vi "List_Files.vi"(8 "error in (no error)":errorcluster, 11 "IB_Source_Container in":refnum<class "IB_Source_Container.lvclass">) -> (0 "error out":errorcluster, 3 "Files":T1[](array[typedef]))   [LabVIEW 2020, in "IB_Source_Container.lvclass"]
uses:
  <vilib>/AppBuilder/IB_Classes/Source/Container/IB_Source_Container.lvclass
  <vilib>/AppBuilder/IB_Classes/Source/Container/IB_Source_Container.lvclass/IB_Source_Container.ctl
  <vilib>/AppBuilder/IB_Classes/Source/IB_Source.lvclass
  <vilib>/AppBuilder/IB_Classes/Source/File/IB_Source_File.lvclass
  <resource>/Framework/Providers/Builds/Installer/CDK_sTypeDef_FileList.ctl
  e:/builds/penguin/labview/branches/2020/dev/dist/vi.lib/AppBuilder/IB_Classes/Source/IB_Source.lvclass
  e:/builds/penguin/labview/branches/2020/dev/dist/vi.lib/AppBuilder/IB_Classes/Source/Container/IB_Source_Container.lvclass
  <vilib>/AppBuilder/IB_Classes/Source/File/CtrFile/IB_CtrFile.lvclass
  e:/builds/penguin/labview/branches/2020/dev/dist/vi.lib/AppBuilder/IB_Classes/Source/File/IB_Source_File.lvclass
  e:/builds/penguin/labview/branches/2020/dev/dist/vi.lib/AppBuilder/IB_Classes/Source/File/CtrFile/IB_CtrFile.lvclass
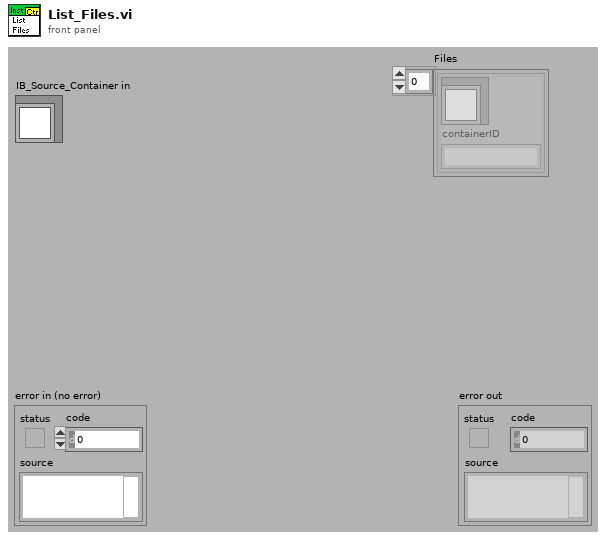
[diagram p1: front panel]
types:
  T1 = typedef "CDK_sTypeDef_FileList.ctl" = cluster{"FileInventory":refnum<class "IB_Source_File.lvclass">, "containerID":string}
  T2 = typedef "IB_Source.ctl" = cluster{"name":string, "sourceTag":string, "destTag":string, "path":path, "eng_installPath":string, "UI_inBuild?":bool, "str ref?":bool}
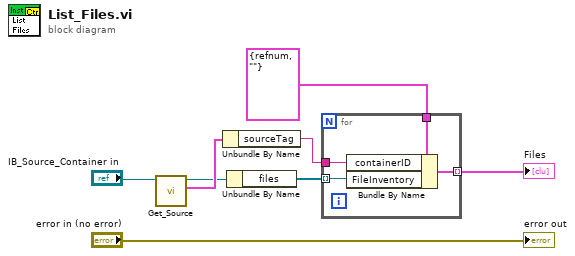
[diagram p0: block diagram]
diagram:
  n1 = call <vilib>:"Get_Source.vi"("IB_Source in"="IB_Source_Container in") -> ("data"=w7:T2, "IB_Source out"=w1:refnum<class "IB_Source_Container.lvclass">)  [unwired: 1 in, 8 out]
  n2 = Unbundle By Name(w7) -> ("sourceTag"=w4:string)
  n3 = Unbundle By Name(w1) -> ("files"=w6:refnum<class "IB_CtrFile.lvclass">[])
  n4 = for {
    tunnel: w6 -> [w11] mode=indexing
    tunnel: T1 {"FileInventory"=refnum, "containerID"=""} ("FileInventory") -> [w12]
    tunnel: w4 -> [w10]
    tunnel: [w9] -> w3 mode=indexing
    n5 = Bundle By Name(cluster=w12, "containerID"=w10, "FileInventory"=w11) -> (w9:T1)
  }
  "Files" <- w3
  "error out" <- "error in (no error)"
